vi "VectorAngle.vi"() -> ()   [LabVIEW 2014]
panel:
  in  "First Point":cluster{"magnitude":dbl, "phase":dbl}
  in  "Second Point":cluster{"magnitude":dbl, "phase":dbl}
  in  "Middle Point":cluster{"magnitude":dbl, "phase":dbl}
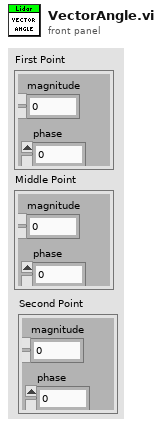
[diagram p1: front panel]
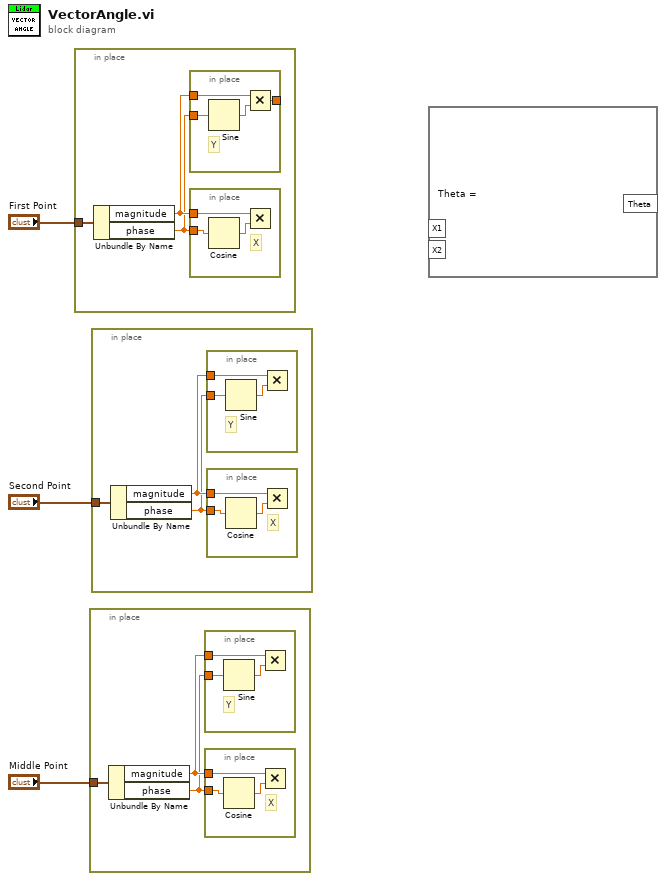
[diagram p0: block diagram]
diagram:
  n1 = in-place {
    in-place-border: "First Point" -> [w6]
    n2 = Unbundle By Name(w6) -> ("magnitude"=w5:dbl, "phase"=w4:dbl)
    n3 = in-place {
      in-place-border: w5 -> [w10]
      in-place-border: w4 -> [w9]
      in-place-border: [w7] -> _
      # "Y"
      n4 = Sine(x=w9) -> (sin(x)=w8:dbl)
      n5 = Multiply(x=w10, y=w8) -> (x*y=w7:dbl)
    }
    n6 = in-place {
      in-place-border: w5 -> [w12]
      in-place-border: w4 -> [w11]
      # "X"
      n7 = Cosine(x=w11) -> (cos(x)=w13:dbl)
      n8 = Multiply(x=w12, y=w13) -> ()  [unwired: 1 out]
    }
  }
  n9 = in-place {
    in-place-border: "Middle Point" -> [w16]
    n10 = Unbundle By Name(w16) -> ("magnitude"=w15:dbl, "phase"=w14:dbl)
    n11 = in-place {
      in-place-border: w15 -> [w19]
      in-place-border: w14 -> [w18]
      # "Y"
      n12 = Sine(x=w18) -> (sin(x)=w17:dbl)
      n13 = Multiply(x=w19, y=w17) -> ()  [unwired: 1 out]
    }
    n14 = in-place {
      in-place-border: w15 -> [w21]
      in-place-border: w14 -> [w20]
      # "X"
      n15 = Cosine(x=w20) -> (cos(x)=w22:dbl)
      n16 = Multiply(x=w21, y=w22) -> ()  [unwired: 1 out]
    }
  }
  n17 = in-place {
    in-place-border: "Second Point" -> [w25]
    n18 = Unbundle By Name(w25) -> ("magnitude"=w24:dbl, "phase"=w23:dbl)
    n19 = in-place {
      in-place-border: w24 -> [w28]
      in-place-border: w23 -> [w27]
      # "Y"
      n20 = Sine(x=w27) -> (sin(x)=w26:dbl)
      n21 = Multiply(x=w28, y=w26) -> ()  [unwired: 1 out]
    }
    n22 = in-place {
      in-place-border: w24 -> [w30]
      in-place-border: w23 -> [w29]
      # "X"
      n23 = Cosine(x=w29) -> (cos(x)=w31:dbl)
      n24 = Multiply(x=w30, y=w31) -> ()  [unwired: 1 out]
    }
  }
  n25 = formula code="Theta ="() -> ()  [unwired: 2 in, 1 out]
